vi "PicoScopeospaSetupStreaming.vi"(0 "handle in":i16=16384, 1 "Streaming Acquisition Settings":T5={"preTriggerSamples"=0, "postTriggerSamples"=10000000, "Requested sampleInterval"=10.0, "sampleIntervalTimeUnits"=2} {"sampleIntervalTimeUnits" items=["femtoseconds", "picoseconds", "nanoseconds", "microseconds", "millseconds", "seconds"]; "postTriggerSamples" format="%_6p"; "preTriggerSamples" format="%_6p"}, 2 "Buffer and Transfer Settings":T4={"startIndex"=0, "Samples"=10000000, "Down Sample Ratio"=1, "Down-Sample Mode"=2147483648} {"Down-Sample Mode" items=["RAW none"=2147483648, "None"=0, "Aggregate"=1, "Decimate"=2, "Average"=4]; "Down Sample Ratio" step=1; "Samples" format="%_6p"}, 3 "enabled array":i16[](array[numeric])=[1, 0, 0, 0, 0, 0, 0, 0, 0, 0], 5 "Device Info":T1={"PICO_DRIVER_VERSION"="", "PICO_USB_VERSION"="", "PICO_HARDWARE_VERSION"="", "PICO_VARIANT_INFO"="", "PICO_BATCH_AND_SERIAL"="", "PICO_CAL_DATE"="", "PICO_KERNEL_VERSION"="", "PICO_DIGITAL_HARDWARE_VERSION"="", "PICO_ANALOGUE_HARDWARE_VERSION"="", "PICO_FIRMWARE_VERSION_1"="", "PICO_FIRMWARE_VERSION_2"="", "PICO_IPP_VERSION"="", "PICO_DRIVER_PATH"="", "PICO_FIRMWARE_VERSION_3"="0", "PICO_FRONT_PANEL_FIRMWARE_VERSION"="0", "Number of Channels"=0, "MSO"=TRUE}, 7 "Data Pointers In":T2={"Max Buffer Pointers"=[[[140687852109952, 80000000], [0, 55], [0, 55], [0, 55], [0, 55], [0, 55], [0, 55], [0, 55], [0, 55], [0, 55]], [[140687772090496, 80000000], [0, 55], [0, 55], [0, 55], [0, 55], [0, 55], [0, 55], [0, 55], [0, 55], [0, 55]]], "Min Buffer Pointers"=[[[0, 0], [0, 77], [0, 77], [0, 77], [0, 77], [0, 77], [0, 77], [0, 77], [0, 77], [0, 77]], [[0, 0], [0, 77], [0, 77], [0, 77], [0, 77], [0, 77], [0, 77], [0, 77], [0, 77], [0, 77]]], "StreamingDataInfo"=[[{"Channel"=0, "Down-Sample Mode"=0, "PICO_DATA_TYPE"=enum."PICO_INT16_T", "Samples"=0, "bufferIndex"=0, "startIndex"=0, "overflow"=0}], [{"Channel"=0, "Down-Sample Mode"=0, "PICO_DATA_TYPE"=enum."PICO_INT8_T", "Samples"=0, "bufferIndex"=0, "startIndex"=0, "overflow"=0}]]}, 9 "Number of Buffers":i32=3, 11 "error in (no error)":errorcluster, 12 "Auto Stop":bool) -> (4 "handle out":i16=16384, 8 "Data Pointers":T2={"Max Buffer Pointers"=[[[140687852109952, 80000000], [0, 55], [0, 55], [0, 55], [0, 55], [0, 55], [0, 55], [0, 55], [0, 55], [0, 55]], [[140687772090496, 80000000], [0, 55], [0, 55], [0, 55], [0, 55], [0, 55], [0, 55], [0, 55], [0, 55], [0, 55]], [[140687231811712, 80000000], [0, 55], [0, 55], [0, 55], [0, 55], [0, 55], [0, 55], [0, 55], [0, 55], [0, 55]]], "Min Buffer Pointers"=[[[0, 0], [0, 77], [0, 77], [0, 77], [0, 77], [0, 77], [0, 77], [0, 77], [0, 77], [0, 77]], [[0, 0], [0, 77], [0, 77], [0, 77], [0, 77], [0, 77], [0, 77], [0, 77], [0, 77], [0, 77]], [[0, 0], [0, 77], [0, 77], [0, 77], [0, 77], [0, 77], [0, 77], [0, 77], [0, 77], [0, 77]]], "StreamingDataInfo"=[[{"Channel"=0, "Down-Sample Mode"=0, "PICO_DATA_TYPE"=enum."PICO_INT16_T", "Samples"=0, "bufferIndex"=0, "startIndex"=0, "overflow"=0}], [{"Channel"=0, "Down-Sample Mode"=0, "PICO_DATA_TYPE"=enum."PICO_INT8_T", "Samples"=0, "bufferIndex"=0, "startIndex"=0, "overflow"=0}], [{"Channel"=0, "Down-Sample Mode"=0, "PICO_DATA_TYPE"=enum."PICO_INT8_T", "Samples"=0, "bufferIndex"=0, "startIndex"=0, "overflow"=0}]]}, 13 "Actual sampleInterval":T3={"sampleInterval"=10.0, "sampleIntervalTimeUnits"=2} {"sampleIntervalTimeUnits" items=["femtoseconds", "picoseconds", "nanoseconds", "microseconds", "millseconds", "seconds", ""]}, 15 "error out":errorcluster)   [LabVIEW 2010]
doc: "Setup streaming Pico data buffers and first calls to SetDataDataBuffer"
uses:
  shared/PicoBuffers.ctl
  psospa.dll
  shared/Buffer and Transfer Settings.ctl
panel:
  in  "Dummy enabled array":i16[](array[numeric])=[1, 1, 1, 1, 1, 1, 1, 1, 1, 1]
  out "Actionflag":bool=TRUE
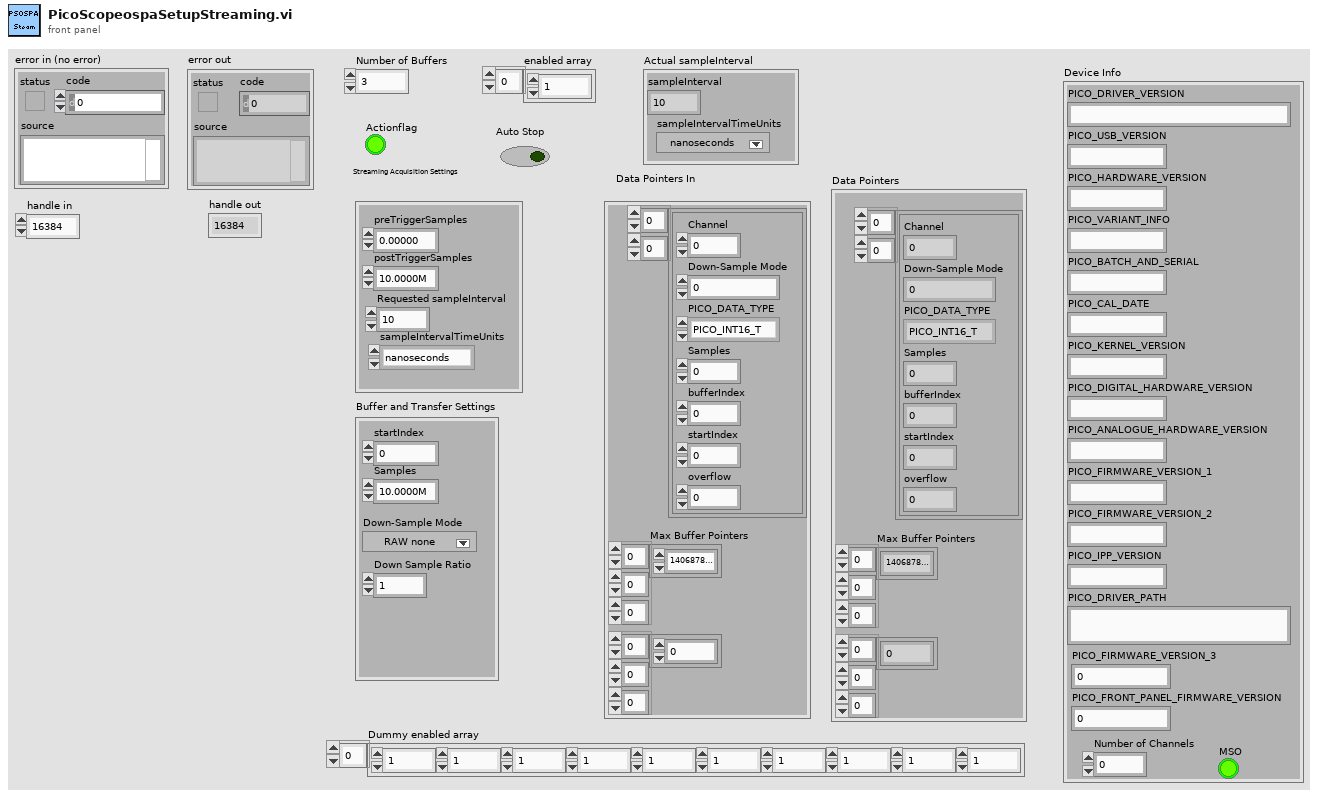
[diagram p1: front panel]
types:
  T1 = cluster{"PICO_DRIVER_VERSION":string, "PICO_USB_VERSION":string, "PICO_HARDWARE_VERSION":string, "PICO_VARIANT_INFO":string, "PICO_BATCH_AND_SERIAL":string, "PICO_CAL_DATE":string, "PICO_KERNEL_VERSION":string, "PICO_DIGITAL_HARDWARE_VERSION":string, "PICO_ANALOGUE_HARDWARE_VERSION":string, "PICO_FIRMWARE_VERSION_1":string, "PICO_FIRMWARE_VERSION_2":string, "PICO_IPP_VERSION":string, "PICO_DRIVER_PATH":string, "PICO_FIRMWARE_VERSION_3":string, "PICO_FRONT_PANEL_FIRMWARE_VERSION":string, "Number of Channels":i16, "MSO":bool}
  T2 = typedef "PicoBuffers.ctl" = cluster{"Max Buffer Pointers":u64[][][], "Min Buffer Pointers":u64[][][], "StreamingDataInfo":cluster{"Channel":u32, "Down-Sample Mode":u32, "PICO_DATA_TYPE":enum32{"PICO_INT8_T", "PICO_INT16_T", "PICO_INT32_T", "PICO_UINT32_T", "PICO_INT64_T", ""}, "Samples":i32, "bufferIndex":u64, "startIndex":i32, "overflow":i16}[][]}
  T3 = cluster{"sampleInterval":dbl, "sampleIntervalTimeUnits":u32}
  T4 = typedef "Buffer and Transfer Settings.ctl" = cluster{"startIndex":u64, "Samples":u64, "Down Sample Ratio":u64, "Down-Sample Mode":u32}
  T5 = cluster{"preTriggerSamples":u64, "postTriggerSamples":u64, "Requested sampleInterval":dbl, "sampleIntervalTimeUnits":u32}
  T6 = cluster{"Channel":u32, "Down-Sample Mode":u32, "PICO_DATA_TYPE":enum32{"PICO_INT8_T", "PICO_INT16_T", "PICO_INT32_T", "PICO_UINT32_T", "PICO_INT64_T", ""}, "Samples":i32, "bufferIndex":u64, "startIndex":i32, "overflow":i16}
  T7 = enum32{"PICO_INT8_T", "PICO_INT16_T", "PICO_INT32_T", "PICO_UINT32_T", "PICO_INT64_T", ""}
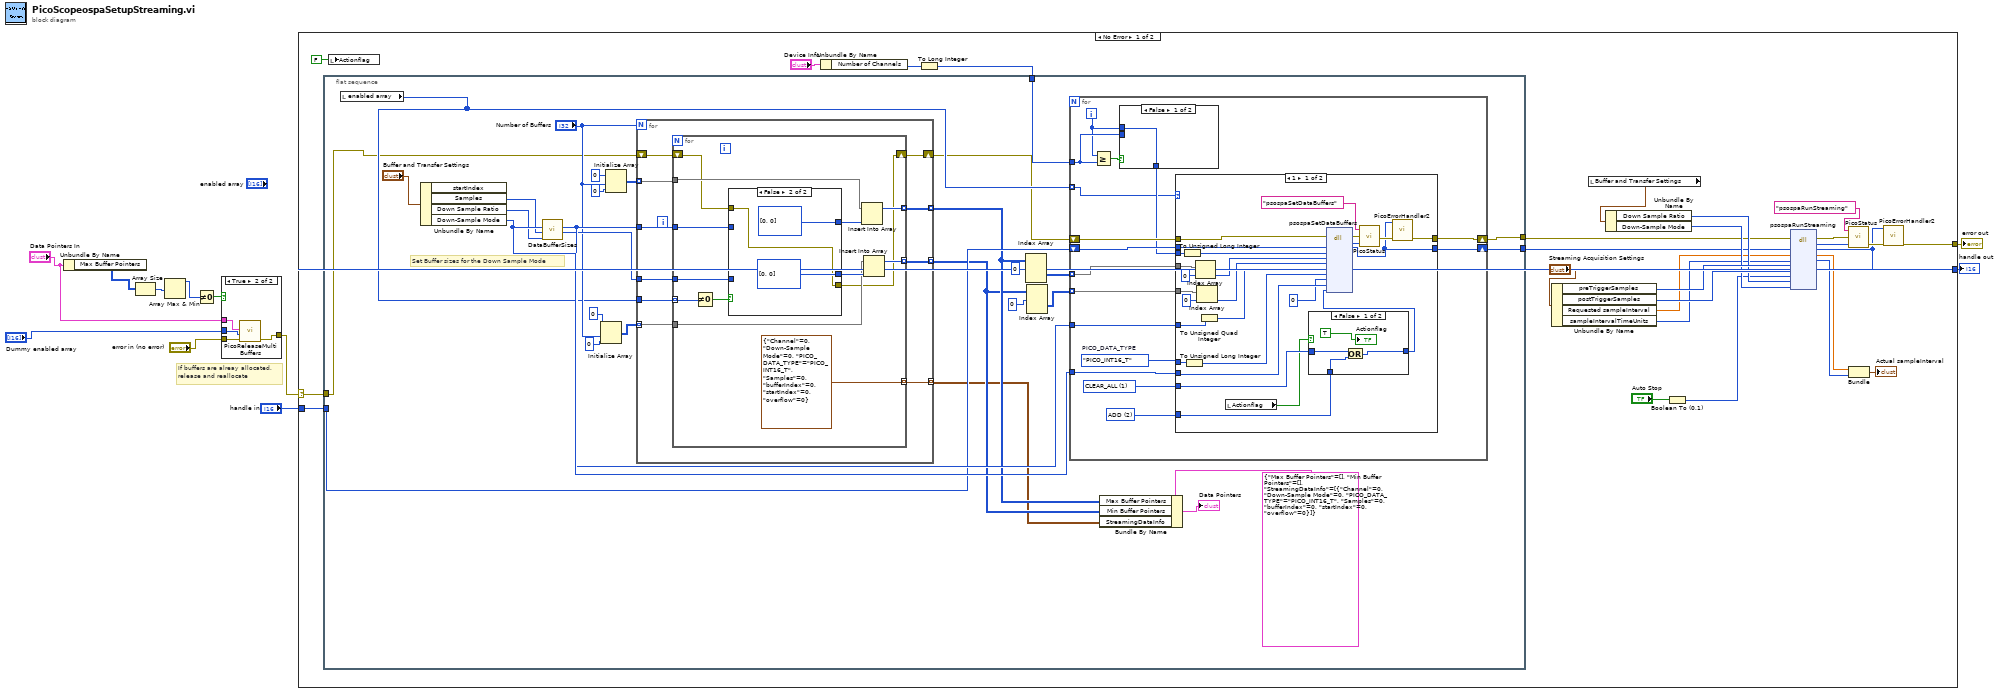
[diagram p0: block diagram]
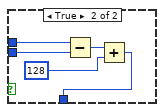
[diagram p3: hidden frame]
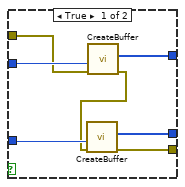
[diagram p6: hidden frame]
diagram:
  # "If buffers are alreay allocated,\nrelease and reallocate"
  n1 = Unbundle By Name("Data Pointers In") -> ("Max Buffer Pointers"=w3:u64[][][])
  n2 = Array Size(array=w3) -> (size(s)=w7:i32[])
  n3 = Array Max & Min(array=w7) -> (max value=w6:i32)  [unwired: 3 out]
  n4 = Not Equal To 0?(x=w6) -> (x != 0?=w8:bool)
  n5 = case shown="True" w8 {
    tunnel: "error in (no error)" -> [w12 w16]
    tunnel: [w12 w15] -> w4
    tunnel: "Dummy enabled array" -> [_ w14]
    tunnel: "Data Pointers In" -> [_ w13]
    frame False {
    }
    frame True {
      n6 = call "PicoReleaseMultiBuffers.vi"("error in (no error)"=w16, "Enabled array"=w14, "Data Pointers"=w13) -> ("error out"=w15:errorcluster)  [unwired: 7 in, 1 out]
    }
  }
  n7 = case shown="No Error" w4 {
    selector: w4 -> [w33 w161]
    tunnel: "handle in" -> [w32 w162]
    tunnel: [w25 w162] -> w10
    tunnel: [w26 w161] -> w9
    frame No Error {
      n8 = flat-sequence {
        tunnel: w33 -> [w45]
        tunnel: w32 -> [w56]
        tunnel: [w57] -> w31
        tunnel: [w53] -> w30
        tunnel: w18 -> [w47]
        frame #0 {
          # "Set Buffer sizes for the Down Sample Mode"
          n9 = local read "enabled array"() -> (w48:i16[])
          n10 = Unbundle By Name("Buffer and Transfer Settings") -> ("Samples"=w65:u64, "Down Sample Ratio"=w64:u64, "Down-Sample Mode"=w66:u32)  [unwired: 1 out]
          n11 = call "DataBufferSizes.vi"("Down Sample Ratio"=w64, "Number of Samples"=w65, "Down-Sample Mode"=w66) -> ("min Buffer Size"=w62:i32, "Max Buffer Size"=w63:i32)  [unwired: 7 in]
          n12 = Initialize Array(u64 0 ("element"), "Number of Buffers", 0 ("dimension size")) -> (w59:u64[][])
          n13 = Initialize Array(u64 0 ("element"), "Number of Buffers", 0 ("dimension size")) -> (w67:u64[][])
          n14 = for {
            N: "Number of Buffers" -> [_]
            tunnel: w48 -> [w136]
            tunnel: w63 -> [w137]
            tunnel: w62 -> [w135]
            tunnel: [w134] -> w52 mode=indexing
            tunnel: w67 -> [w133] mode=indexing
            tunnel: w59 -> [w132] mode=indexing
            tunnel: [w131] -> w51 mode=indexing
            tunnel: [w130] -> w46 mode=indexing
            shift-right: [w128] -> w44
            shift-left: w45 -> [w129]
            n15 = for {
              tunnel: w137 -> [w150]
              tunnel: w136 -> [w148] mode=indexing
              tunnel: w135 -> [w147]
              tunnel: [w145] -> w134 mode=indexing
              tunnel: w133 -> [w144]
              tunnel: w132 -> [w142]
              tunnel: [w141] -> w131 mode=indexing
              tunnel: [T6 {"Channel"=0, "Down-Sample Mode"=0, "PICO_DATA_TYPE"=enum."PICO_INT16_T", "Samples"=0, "bufferIndex"=0, "startIndex"=0, "overflow"=0} ("C Struture define 3")] -> w130 mode=indexing
              shift-right: [w138] -> w128
              shift-left: w129 -> [w139]
              n16 = Not Equal To 0?(x=w148) -> (x != 0?=w149:bool)
              n17 = case shown="False" w149 {
                tunnel: w150 -> [w156 _]
                tunnel: w147 -> [w157 _]
                tunnel: [w155 u64[] [0, 0]] -> w146
                tunnel: [w154 u64[] [0, 0]] -> w143
                tunnel: w139 -> [w153 w158]
                tunnel: [w151 w158] -> w138
                frame True {
                  n18 = call "CreateBuffer.vi"("error in (no error)"=w153, "Buffer size"=w156) -> ("error out"=w152:errorcluster, "Pointer and BufferSize"=w155:u64[])  [unwired: 8 in]
                  n19 = call "CreateBuffer.vi"("error in (no error)"=w152, "Buffer size"=w157) -> ("error out"=w151:errorcluster, "Pointer and BufferSize"=w154:u64[])  [unwired: 8 in]
                }
                frame False {
                }
              }
              n20 = Insert Into Array(array=w144, new element=w146) -> (w145:u64[])  [unwired: 1 in]
              n21 = Insert Into Array(array=w142, new element=w143) -> (w141:u64[])  [unwired: 1 in]
            }
          }
          n22 = Index Array(array=w52, index (dim 0)=0 ("index")) -> (element=w70:u64[][])  [unwired: 2 in]
          n23 = Index Array(array=w51, index (dim 0)=0 ("index")) -> (element=w54:u64[][])  [unwired: 2 in]
          n24 = for {
            tunnel: w66 -> [w88]
            tunnel: w63 -> [w83]
            tunnel: w48 -> [w73] mode=indexing
            tunnel: w70 -> [w82] mode=indexing
            shift-right: [w81] -> w57
            shift-left: w44 -> [w87]
            tunnel: w54 -> [w77] mode=indexing
            shift-right: [w76] -> w53
            shift-left: w56 -> [w86]
            tunnel: w47 -> [w75]
            i -> [w74]
            w78 = T7."PICO_INT16_T"  # PICO_DATA_TYPE
            w79 = u32 1 items=["NONE"=0, "CLEAR_ALL"=1, "ADD"=2, "CLEAR_THIS_DATA_BUFFER"=4096, "CLEAR_WAVEFORM_DATA_BUFFERS"=8192, "CLEAR_WAVEFORM_READ_DATA_BUFFERS"=16384] ("PicoAction 1")
            w80 = u32 2 items=["NONE"=0, "CLEAR_ALL"=1, "ADD"=2, "CLEAR_THIS_DATA_BUFFER"=4096, "CLEAR_WAVEFORM_DATA_BUFFERS"=8192, "CLEAR_WAVEFORM_READ_DATA_BUFFERS"=16384] ("PicoAction 2")
            n25 = Greater Or Equal?(x=w74, y=w75) -> (x >= y?=w85:bool)
            n26 = case shown="False" w85 {
              tunnel: [w89 w93] -> w84
              tunnel: w75 -> [_ w92]
              tunnel: w74 -> [w89 w91]
              frame False {
              }
              frame True {
                n27 = Subtract(x=w91, y=w92) -> (x-y=w90:i32)
                n28 = Add(x=w90, y=128) -> (x+y=w93:i32)
              }
            }
            n29 = case shown="1" w73 {
              tunnel: w84 -> [w109 _]
              tunnel: w87 -> [w120 w127]
              tunnel: w86 -> [w117 w126]
              tunnel: w88 -> [w114 _]
              tunnel: w78 -> [w99 _]
              tunnel: w79 -> [w104 _]
              tunnel: [w113 w127] -> w81
              tunnel: [w112 w126] -> w76
              tunnel: w83 -> [w111 _]
              tunnel: w82 -> [w105 _]
              tunnel: w80 -> [w103 _]
              tunnel: w77 -> [w95 _]
              frame 1 {
                n30 = To Unsigned Long Integer(number=w109) -> (unsigned 32bit integer=w108:u32)
                n31 = To Unsigned Long Integer(number=w99) -> (unsigned 32bit integer=w100:u32)
                n32 = Index Array(array=w105, index=0) -> (element=w106:u64)
                n33 = Index Array(array=w95, index=0) -> (element=w96:u64)
                n34 = To Unsigned Quad Integer(1:w111) -> (0:w110:u64)
                n35 = local read "Actionflag"() -> (w101:bool)
                n36 = case shown="False" w101 {
                  tunnel: w104 -> [w124 _]
                  tunnel: w103 -> [w123 w125]
                  tunnel: [w122 w125] -> w102
                  frame False {
                    n37 = Or(x=w124, y=w123) -> (x .or. y?=w122:u32)
                    "Actionflag" <- TRUE ("Actionflag")
                  }
                  frame True {
                  }
                }
                n38 = dll-call lib="psospa.dll" fn="psospaSetDataBuffers" ("ps3000.dll:_ps3000_open_unit@0")(error in=w120, "handle"=w117, "channel"=w108, "bufferMax"=w106, "bufferMin"=w96, "nSamples"=w110, "dataType"=w100, "waveform"=u64 0, "downSampleRatioMode"=w114, "action"=w102) -> (error out=w119:errorcluster, "PICO_STATUS"=w118:u32, "handle"=w112:i16)  [unwired: 10 in, 1 out]
                n39 = call "PicoStatus.vi"("PICO STATUS"=w118, "error in"=w119, "source"="psospaSetDataBuffers") -> ("error out"=w115:errorcluster)
                n40 = call "PicoErrorHandler2.vi"("error in (no error)"=w115, "handle In"=w112) -> ("error out"=w113:errorcluster)  [unwired: 9 in]
              }
              frame 0, Default {
              }
            }
          }
          n41 = Bundle By Name(cluster=T2 {"Max Buffer Pointers"=[], "Min Buffer Pointers"=[], "StreamingDataInfo"=[[{"Channel"=0, "Down-Sample Mode"=0, "PICO_DATA_TYPE"=enum."PICO_INT16_T", "Samples"=0, "bufferIndex"=0, "startIndex"=0, "overflow"=0}]]} ("Data Pointers"), "Max Buffer Pointers"=w52, "Min Buffer Pointers"=w51, "StreamingDataInfo"=w46) -> (→"Data Pointers":T2)
        }
      }
      n42 = local write "Actionflag"(FALSE ("Actionflag")) -> ()
      n43 = Unbundle By Name("Device Info") -> ("Number of Channels"=w17:i16)
      n44 = To Long Integer(number=w17) -> (32bit integer=w18:i32)
      n45 = Unbundle By Name("Streaming Acquisition Settings") -> ("preTriggerSamples"=w38:u64, "postTriggerSamples"=w37:u64, "Requested sampleInterval"=w29:dbl, "sampleIntervalTimeUnits"=w28:u32)
      n46 = local read "Buffer and Transfer Settings"() -> (w36:T4)
      n47 = Unbundle By Name(w36) -> ("Down Sample Ratio"=w35:u64, "Down-Sample Mode"=w34:u32)
      n48 = Boolean To (0,1)(Boolean="Auto Stop") -> (0, 1=w20:i16)
      n49 = dll-call lib="psospa.dll" fn="psospaRunStreaming" ("ps3000.dll:_ps3000_open_unit@0")(error in=w31, "handle"=w30, "sampleInterval"=w29, "sampleIntervalTimeUnits"=w28, "maxPreTriggerSamples"=w38, "maxPostPreTriggerSamples"=w37, "autoStop"=w20, "downSampleRatio"=w35, "downSampleRatioMode"=w34) -> (error out=w42:errorcluster, "PICO_STATUS"=w41:u32, "handle"=w25:i16, "sampleInterval"=w24:dbl, "sampleIntervalTimeUnits"=w23:u32)  [unwired: 7 in, 1 out]
      n50 = call "PicoStatus.vi"("PICO STATUS"=w41, "error in"=w42, "source"="psospaRunStreaming") -> ("error out"=w43:errorcluster)
      n51 = Bundle("sampleInterval"=w24, "sampleIntervalTimeUnits"=w23) -> (→"Actual sampleInterval":T3)  [unwired: 1 in]
      n52 = call "PicoErrorHandler2.vi"("error in (no error)"=w43, "handle In"=w25) -> ("error out"=w26:errorcluster)  [unwired: 9 in]
    }
    frame Error {
    }
  }
  "handle out" <- w10
  "error out" <- w9
